vi "Read and Write Text File.vi"(8 "error in (no error)":errorcluster, 11 "Byte Stream File in":refnum<file>) -> (0 "error out":errorcluster, 3 "Byte Stream File out":refnum<file>)   [LabVIEW 2015]
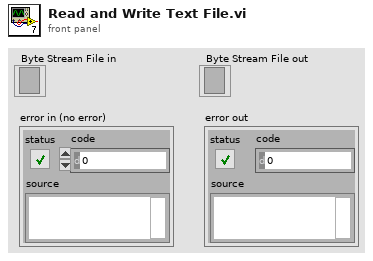
[diagram p1: front panel]
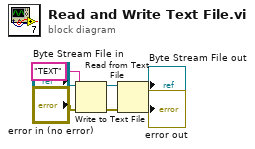
[diagram p0: block diagram]
diagram:
  n1 = Write to Text File(file (use dialog)="Byte Stream File in", text="TEXT", error in="error in (no error)") -> (refnum out=w3:refnum<file>, error out=w4:errorcluster)  [unwired: 1 in, 1 out]
  n2 = Read from Text File(file (use dialog)=w3, error in=w4) -> (refnum out=→"Byte Stream File out":refnum<file>, error out=→"error out":errorcluster)  [unwired: 2 in, 2 out]
